vi "Stop.vi"(8 "error in":errorcluster, 11 "Red-y Read Write CFG in":refnum<class "Red-y Pressure Control CFG.lvclass">) -> (0 "error out":errorcluster, 3 "Red-y Read Write CFG out":refnum<class "Red-y Pressure Control CFG.lvclass">)   [LabVIEW 2023, in "Red-y Pressure Control CFG.lvclass"]
uses:
  Red-y Pressure Control CFG.lvclass
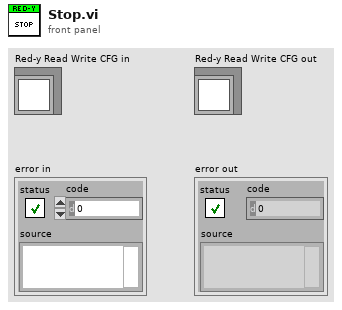
[diagram p1: front panel]
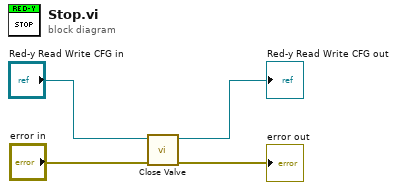
[diagram p0: block diagram]
diagram:
  n1 = call-dynamic "Close Valve.vi"("error in"="error in", "Red-y Read Write CFG in"="Red-y Read Write CFG in") -> ("error out"=→"error out":errorcluster, "Red-y Read Write CFG out"=→"Red-y Read Write CFG out":refnum<class "Red-y Pressure Control CFG.lvclass">)  [unwired: 8 in]
